vi "DataToJson.vi"(1 "Array":string[][](array[string])) -> (0 "Json":string)   [LabVIEW 2019]
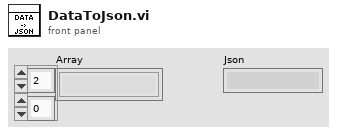
[diagram p1: front panel]
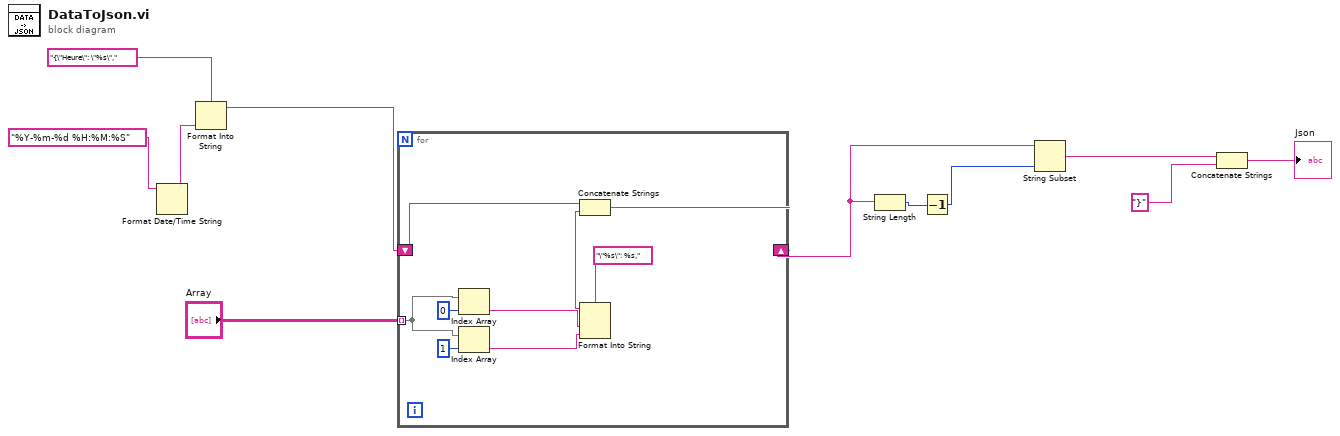
[diagram p0: block diagram]
diagram:
  n1 = Format Date/Time String(time format string (%c)="%Y-%m-%d %H:%M:%S") -> (date/time string=w2:string)  [unwired: 2 in]
  n2 = Format Into String(format string="{\"Heure\": \"%s\",", w2) -> (resulting string=w10:string)  [unwired: 2 in, 1 out]
  n3 = for {
    shift-right: [w19] -> w5
    shift-left: w10 -> [w20]
    tunnel: "Array" -> [w16] mode=indexing
    n4 = Index Array(array=w16, index=0) -> (element=w14:string)
    n5 = Index Array(array=w16, index=1) -> (element=w13:string)
    n6 = Format Into String(format string="\"%s\": %s,", w14, w13) -> (resulting string=w12:string)  [unwired: 2 in, 1 out]
    n7 = Concatenate Strings(w20, w12) -> (w19:string)
  }
  n8 = String Length(string=w5) -> (length=w7:i32)
  n9 = Decrement(x=w7) -> (x-1=w6:i32)
  n10 = String Subset(string=w5, length (rest)=w6) -> (substring=w4:string)  [unwired: 1 in]
  n11 = Concatenate Strings(w4, "}" ("string")) -> (→"Json":string)
